vi "Handle Endianity.vi"(8 "error in (no error)":errorcluster, 10 "Byte to read in":string, 11 "TCP Text Listener in":refnum<class "TCP Text Listener.lvclass">) -> (0 "error out":errorcluster, 2 "Bytes to read out":string, 3 "TCP Text Listener out":refnum<class "TCP Text Listener.lvclass">)   [LabVIEW 2026, in "TALOS.lvlib" / "TCP Text Listener.lvlib" / "TCP Text Listener.lvclass"]
uses:
  TCP Text Listener.lvclass
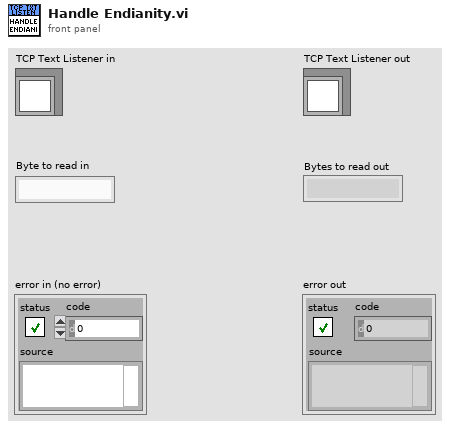
[diagram p1: front panel]
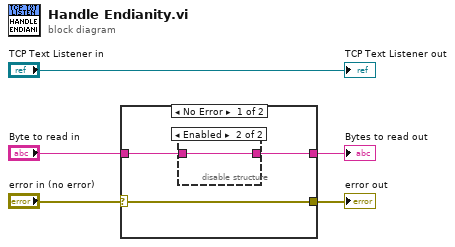
[diagram p0: block diagram]
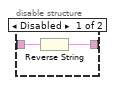
[diagram p2: hidden frame]
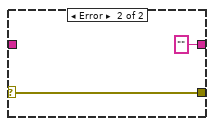
[diagram p3: hidden frame]
diagram:
  n1 = case shown="No Error" "error in (no error)" {
    selector: "error in (no error)" -> [w8 w13]
    tunnel: [w8 w13] -> w4
    tunnel: [w6 "" ("Byte to read in")] -> w2
    tunnel: "Byte to read in" -> [w7 _]
    frame No Error {
      n2 = disable-structure shown="Enabled" {
        disable-tunnel: w7 -> [w10 w11]
        disable-tunnel: [w9 w11] -> w6
        frame Disabled {
          n3 = Reverse String(1:w10) -> (0:w9:string)
        }
        frame Enabled {
        }
      }
    }
    frame Error {
    }
  }
  "error out" <- w4
  "Bytes to read out" <- w2
  "TCP Text Listener out" <- "TCP Text Listener in"
